vi "Transfer_function_diagonal_2register.vi"(0 "X reference":fxp<+/-,32,16>, 1 "Y reference":fxp<+/-,32,16>, 2 "Z reference":fxp<+/-,32,16>, 3 "X actual":fxp<+/-,33,17>, 4 "Y actual":fxp<+/-,33,17>, 5 "Z actual":fxp<+/-,33,17>, 6 "Scaling mV to V":fxp<+,33,10>=0.0009765625, 7 "xx1 Transfer Function":T1={"sos gain SF Controller"=0.0, "-a01(2)"=[0.0, 0.0, 0.0, 0.0, 0.0, 0.0, 0.0, 0.0, 0.0, 0.0, 0.0, 0.0, 0.0, 0.0, 0.0, 0.0, 0.0, 0.0, 0.0, 0.0], "-a02(2)"=[0.0, 0.0, 0.0, 0.0, 0.0, 0.0, 0.0, 0.0, 0.0, 0.0, 0.0, 0.0, 0.0, 0.0, 0.0, 0.0, 0.0, 0.0, 0.0, 0.0], "b01(2)"=[0.0, 0.0, 0.0, 0.0, 0.0, 0.0, 0.0, 0.0, 0.0, 0.0, 0.0, 0.0, 0.0, 0.0, 0.0, 0.0, 0.0, 0.0, 0.0, 0.0], "b02(2)"=[0.0, 0.0, 0.0, 0.0, 0.0, 0.0, 0.0, 0.0, 0.0, 0.0, 0.0, 0.0, 0.0, 0.0, 0.0, 0.0, 0.0, 0.0, 0.0, 0.0]}, 8 "Action":T2, 9 "yy1 Transfer Function":T1={"sos gain SF Controller"=0.0, "-a01(2)"=[0.0, 0.0, 0.0, 0.0, 0.0, 0.0, 0.0, 0.0, 0.0, 0.0, 0.0, 0.0, 0.0, 0.0, 0.0, 0.0, 0.0, 0.0, 0.0, 0.0], "-a02(2)"=[0.0, 0.0, 0.0, 0.0, 0.0, 0.0, 0.0, 0.0, 0.0, 0.0, 0.0, 0.0, 0.0, 0.0, 0.0, 0.0, 0.0, 0.0, 0.0, 0.0], "b01(2)"=[0.0, 0.0, 0.0, 0.0, 0.0, 0.0, 0.0, 0.0, 0.0, 0.0, 0.0, 0.0, 0.0, 0.0, 0.0, 0.0, 0.0, 0.0, 0.0, 0.0], "b02(2)"=[0.0, 0.0, 0.0, 0.0, 0.0, 0.0, 0.0, 0.0, 0.0, 0.0, 0.0, 0.0, 0.0, 0.0, 0.0, 0.0, 0.0, 0.0, 0.0, 0.0]}, 11 "zz1 Transfer Function":T1={"sos gain SF Controller"=0.0, "-a01(2)"=[0.0, 0.0, 0.0, 0.0, 0.0, 0.0, 0.0, 0.0, 0.0, 0.0, 0.0, 0.0, 0.0, 0.0, 0.0, 0.0, 0.0, 0.0, 0.0, 0.0], "-a02(2)"=[0.0, 0.0, 0.0, 0.0, 0.0, 0.0, 0.0, 0.0, 0.0, 0.0, 0.0, 0.0, 0.0, 0.0, 0.0, 0.0, 0.0, 0.0, 0.0, 0.0], "b01(2)"=[0.0, 0.0, 0.0, 0.0, 0.0, 0.0, 0.0, 0.0, 0.0, 0.0, 0.0, 0.0, 0.0, 0.0, 0.0, 0.0, 0.0, 0.0, 0.0, 0.0], "b02(2)"=[0.0, 0.0, 0.0, 0.0, 0.0, 0.0, 0.0, 0.0, 0.0, 0.0, 0.0, 0.0, 0.0, 0.0, 0.0, 0.0, 0.0, 0.0, 0.0, 0.0]}) -> (14 "X-stage voltage":fxp<+/-,32,16>, 15 "Y-stage voltage":fxp<+/-,32,16>, 16 "Z-stage voltage":fxp<+/-,32,16>, 17 "Kxx Output, Kxx*ex (V)":fxp<+/-,58,25>, 18 "Kyy Output, Kyy*ey (V)":fxp<+/-,58,25>, 19 "Kzz Output, Kzz*ez (V)":fxp<+/-,58,25>)   [LabVIEW 2015]
uses:
  Transfer_function_actions.ctl
  Transfer_function_coeffs.ctl
  <vilib>/rvi/Emulation/niFpgaGetClockAttributes.vi
  <vilib>/rvi/Emulation/niFpgaSctlEmulationGetInTimedLoop.vi
  <vilib>/rvi/Emulation/niFpgaEmulationReportErrorSimple.vi
  <vilib>/rvi/Emulation/niFpgaCriticalErrorInLSC.vi
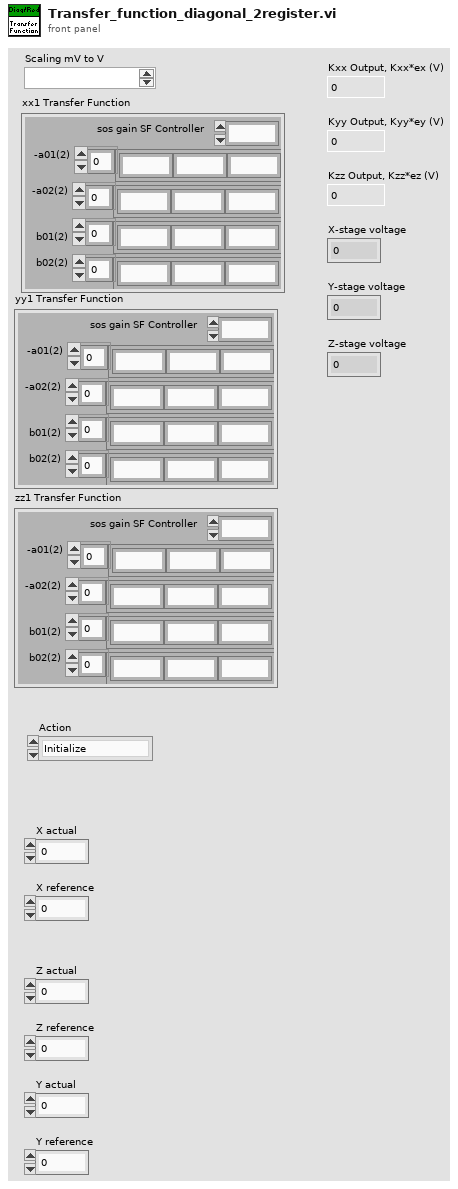
[diagram p1: front panel]
types:
  T1 = typedef "Transfer_function_coeffs.ctl" = cluster{"sos gain SF Controller":fxp<+/-,42,9>, "-a01(2)":fxp<+/-,64,9>[], "-a02(2)":fxp<+/-,64,9>[], "b01(2)":fxp<+/-,64,9>[], "b02(2)":fxp<+/-,64,9>[]}
  T2 = typedef "Transfer_function_actions.ctl" = enum16{"Initialize", "Calculate"}
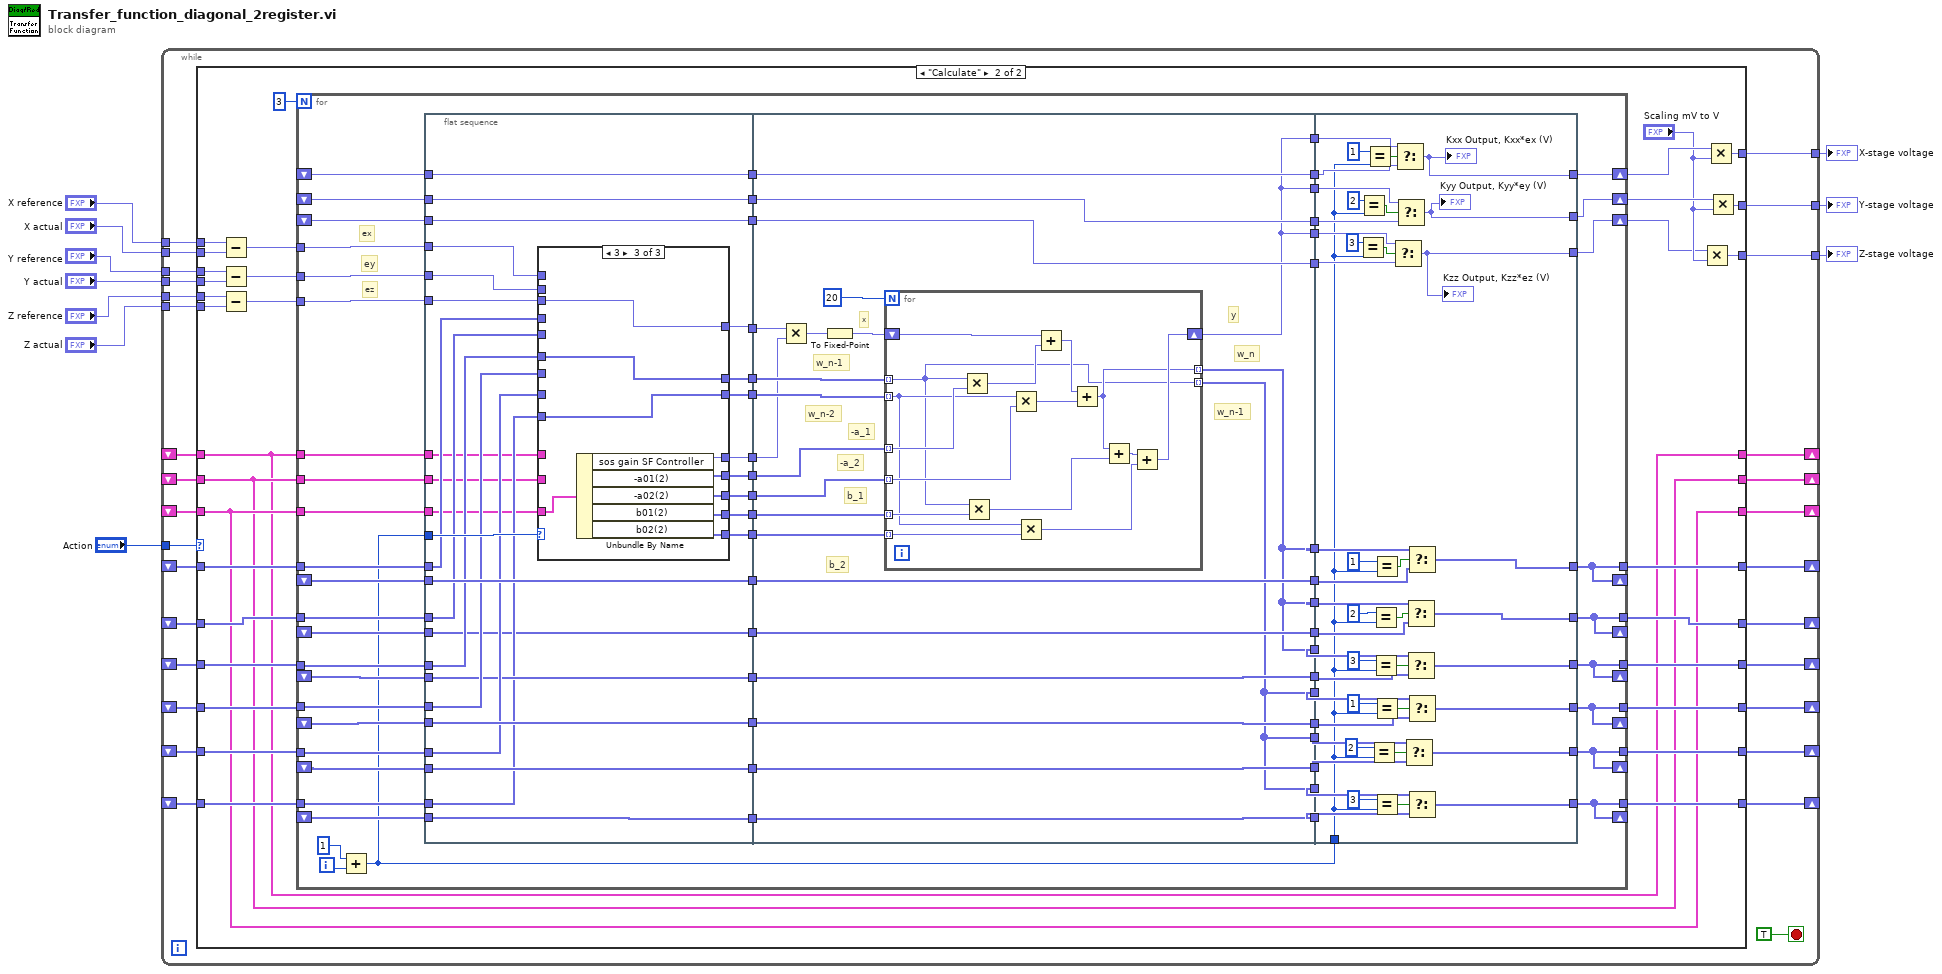
[diagram p0: block diagram]
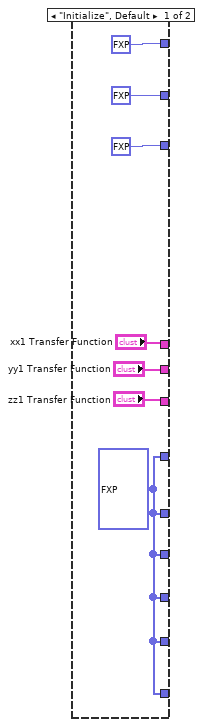
[diagram p2: hidden frame]
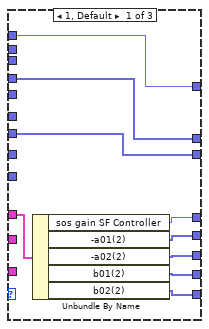
[diagram p3: hidden frame]
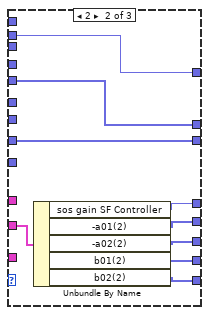
[diagram p4: hidden frame]
diagram:
  n1 = while {
    tunnel: [w39] -> w10
    tunnel: [w38] -> w9
    tunnel: [w37] -> w8
    tunnel: "Z reference" -> [w36]
    tunnel: "Y reference" -> [w35]
    tunnel: "X reference" -> [w34]
    tunnel: "Z actual" -> [w33]
    tunnel: "Y actual" -> [w32]
    tunnel: "X actual" -> [w31]
    shift-right: [w30] -> _
    shift-left: _ -> [w24]
    shift-right: [w29] -> _
    shift-left: _ -> [w23]
    shift-right: [w28] -> _
    shift-left: _ -> [w22]
    shift-right: [w27] -> _
    shift-left: _ -> [w21]
    shift-right: [w26] -> _
    shift-left: _ -> [w20]
    shift-right: [w25] -> _
    shift-left: _ -> [w19]
    tunnel: "Action" -> [w17]
    shift-right: [w13] -> _
    shift-left: _ -> [w16]
    shift-right: [w12] -> _
    shift-left: _ -> [w15]
    shift-right: [w11] -> _
    shift-left: _ -> [w14]
    stop <- TRUE stop-if-true
    n2 = case shown="\"Calculate\"" w17 {
      tunnel: [fxp<+/-,32,16> 0.0 w78] -> w39
      tunnel: [fxp<+/-,32,16> 0.0 w77] -> w38
      tunnel: [fxp<+/-,32,16> 0.0 w76] -> w37
      tunnel: w36 -> [_ w75]
      tunnel: w35 -> [_ w74]
      tunnel: w34 -> [_ w73]
      tunnel: w33 -> [_ w69]
      tunnel: w32 -> [_ w68]
      tunnel: w31 -> [_ w67]
      tunnel: [w43 w65] -> w30
      tunnel: [w43 w64] -> w29
      tunnel: [w43 w63] -> w28
      tunnel: [w43 w62] -> w27
      tunnel: [w43 w61] -> w26
      tunnel: [w43 w60] -> w25
      tunnel: w24 -> [_ w59]
      tunnel: w23 -> [_ w58]
      tunnel: w22 -> [_ w57]
      tunnel: w21 -> [_ w56]
      tunnel: w20 -> [_ w55]
      tunnel: w19 -> [_ w54]
      tunnel: w16 -> [_ w51]
      tunnel: w15 -> [_ w52]
      tunnel: w14 -> [_ w53]
      tunnel: ["xx1 Transfer Function" w51] -> w13
      tunnel: ["yy1 Transfer Function" w52] -> w12
      tunnel: ["zz1 Transfer Function" w53] -> w11
      frame "Initialize", Default {
        w43 = fxp<+/-,58,25>[] [0.0, 0.0, 0.0, 0.0, 0.0, 0.0, 0.0, 0.0, 0.0, 0.0, 0.0, 0.0, 0.0, 0.0, 0.0, 0.0, 0.0, 0.0, 0.0, 0.0]
      }
      frame "Calculate" {
        n3 = Subtract(x=w73, y=w67) -> (x-y=w50:fxp<+/-,58,25>)
        n4 = Subtract(x=w74, y=w68) -> (x-y=w49:fxp<+/-,58,25>)
        n5 = Subtract(x=w75, y=w69) -> (x-y=w48:fxp<+/-,58,25>)
        n6 = for {
          N: 3 -> [_]
          shift-right: [w132] -> w71
          shift-left: _ -> [w130]
          shift-right: [w129] -> w72
          shift-left: _ -> [w127]
          tunnel: [w84] -> w65
          shift-right: [w84] -> _
          shift-left: _ -> [w121]
          tunnel: [w83] -> w64
          shift-right: [w83] -> _
          shift-left: _ -> [w119]
          tunnel: w59 -> [w116]
          tunnel: w58 -> [w115]
          tunnel: [w81] -> w62
          shift-right: [w81] -> _
          shift-left: _ -> [w114]
          tunnel: [w80] -> w61
          shift-right: [w80] -> _
          shift-left: _ -> [w113]
          tunnel: w56 -> [w112]
          tunnel: w55 -> [w111]
          tunnel: w50 -> [w106]
          tunnel: w49 -> [w105]
          shift-right: [w104] -> w47
          shift-left: _ -> [w101]
          tunnel: [w82] -> w63
          tunnel: [w79] -> w60
          shift-right: [w82] -> _
          shift-left: _ -> [w96]
          shift-right: [w79] -> _
          shift-left: _ -> [w94]
          tunnel: w57 -> [w93]
          tunnel: w54 -> [w92]
          tunnel: w48 -> [w89]
          tunnel: w51 -> [w87]
          tunnel: w52 -> [w86]
          tunnel: w53 -> [w85]
          i -> [w137]
          # "ez"
          # "ey"
          # "ex"
          n7 = Add(x=1, y=w137) -> (x+y=w88:i32)
          n8 = flat-sequence {
            tunnel: [w175] -> w146
            tunnel: [w174] -> w145
            tunnel: [w173] -> w144
            tunnel: [w172] -> w143
            tunnel: [w171] -> w142
            tunnel: [w170] -> w141
            tunnel: [w169] -> w140
            tunnel: w88 -> [w176]
            tunnel: [w159] -> w139
            tunnel: [w168] -> w131
            tunnel: w130 -> [w168]
            tunnel: [w167] -> w128
            tunnel: w127 -> [w167]
            tunnel: [w166] -> w122
            tunnel: w121 -> [w166]
            tunnel: [w153] -> w120
            tunnel: w119 -> [w153]
            tunnel: w116 -> [w160]
            tunnel: w115 -> [w161]
            tunnel: w114 -> [w165]
            tunnel: w113 -> [w164]
            tunnel: w112 -> [w162]
            tunnel: w111 -> [w163]
            tunnel: [w165] -> w110
            tunnel: [w164] -> w109
            tunnel: w106 -> [w152]
            tunnel: w105 -> [w151]
            tunnel: [w158] -> w102
            tunnel: w101 -> [w158]
            tunnel: [w157] -> w97
            tunnel: w96 -> [w157]
            tunnel: [w156] -> w95
            tunnel: w94 -> [w156]
            tunnel: w93 -> [w154]
            tunnel: w92 -> [w155]
            tunnel: w89 -> [w150]
            tunnel: w87 -> [w149]
            tunnel: w86 -> [w148]
            tunnel: w85 -> [w147]
            tunnel: w146 -> [w224]
            tunnel: w145 -> [w223]
            tunnel: w144 -> [w208]
            tunnel: w143 -> [w209]
            tunnel: w142 -> [w210]
            tunnel: w141 -> [w211]
            tunnel: w140 -> [w212]
            tunnel: w139 -> [w215]
            tunnel: [w204] -> w136
            tunnel: [w204] -> w135
            tunnel: [w206] -> w134
            tunnel: [w207] -> w133
            tunnel: w131 -> [w207]
            tunnel: w128 -> [w206]
            tunnel: [w214] -> w126
            tunnel: [w214] -> w125
            tunnel: [w213] -> w124
            tunnel: [w213] -> w123
            tunnel: w122 -> [w222]
            tunnel: w120 -> [w221]
            tunnel: [w222] -> w118
            tunnel: [w221] -> w117
            tunnel: w110 -> [w220]
            tunnel: w109 -> [w219]
            tunnel: [w220] -> w108
            tunnel: [w219] -> w107
            tunnel: [w204] -> w103
            tunnel: w102 -> [w218]
            tunnel: [w218] -> w100
            tunnel: [w214] -> w99
            tunnel: [w213] -> w98
            tunnel: w97 -> [w217]
            tunnel: w95 -> [w216]
            tunnel: [w217] -> w91
            tunnel: [w216] -> w90
            tunnel: w136 -> [w244]
            tunnel: w135 -> [w283]
            tunnel: w88 -> [w243]
            tunnel: w134 -> [w282]
            tunnel: w133 -> [w245]
            tunnel: [w242] -> w132
            tunnel: [w247] -> w129
            tunnel: w126 -> [w273]
            tunnel: w125 -> [w272]
            tunnel: w124 -> [w271]
            tunnel: w123 -> [w270]
            tunnel: [w269] -> w84
            tunnel: [w268] -> w83
            tunnel: w118 -> [w267]
            tunnel: w117 -> [w266]
            tunnel: [w265] -> w81
            tunnel: [w264] -> w80
            tunnel: w108 -> [w263]
            tunnel: w107 -> [w262]
            tunnel: [w246] -> w104
            tunnel: w103 -> [w259]
            tunnel: w100 -> [w258]
            tunnel: w99 -> [w253]
            tunnel: w98 -> [w252]
            tunnel: [w251] -> w82
            tunnel: [w250] -> w79
            tunnel: w91 -> [w249]
            tunnel: w90 -> [w248]
            frame #0 {
              n9 = case shown="3" w176 {
                tunnel: [w182 w190 w199] -> w173
                tunnel: [w181 w189 w198] -> w172
                tunnel: [w180 w188 w197] -> w171
                tunnel: [w179 w187 w196] -> w170
                tunnel: [w178 w186 w195] -> w169
                tunnel: [w183 w193 w202] -> w174
                tunnel: [w184 w192 w201] -> w175
                tunnel: w160 -> [w184 _ _]
                tunnel: w161 -> [_ w192 _]
                tunnel: w162 -> [w183 _ _]
                tunnel: w163 -> [_ w193 _]
                tunnel: [w185 w194 w203] -> w159
                tunnel: w152 -> [w185 _ _]
                tunnel: w151 -> [_ w194 _]
                tunnel: w155 -> [_ _ w202]
                tunnel: w154 -> [_ _ w201]
                tunnel: w150 -> [_ _ w203]
                tunnel: w149 -> [w177 _ _]
                tunnel: w148 -> [_ w191 _]
                tunnel: w147 -> [_ _ w200]
                frame 1, Default {
                  n10 = Unbundle By Name(w177) -> ("sos gain SF Controller"=w182:fxp<+/-,42,9>, "-a01(2)"=w181:fxp<+/-,64,9>[], "-a02(2)"=w180:fxp<+/-,64,9>[], "b01(2)"=w179:fxp<+/-,64,9>[], "b02(2)"=w178:fxp<+/-,64,9>[])
                }
                frame 2 {
                  n11 = Unbundle By Name(w191) -> ("sos gain SF Controller"=w190:fxp<+/-,42,9>, "-a01(2)"=w189:fxp<+/-,64,9>[], "-a02(2)"=w188:fxp<+/-,64,9>[], "b01(2)"=w187:fxp<+/-,64,9>[], "b02(2)"=w186:fxp<+/-,64,9>[])
                }
                frame 3 {
                  n12 = Unbundle By Name(w200) -> ("sos gain SF Controller"=w199:fxp<+/-,42,9>, "-a01(2)"=w198:fxp<+/-,64,9>[], "-a02(2)"=w197:fxp<+/-,64,9>[], "b01(2)"=w196:fxp<+/-,64,9>[], "b02(2)"=w195:fxp<+/-,64,9>[])
                }
              }
            }
            frame #1 {
              # "b_2"
              # "b_1"
              # "-a_2"
              # "-a_1"
              # "w_n-2"
              # "x"
              # "w_n-1"
              # "w_n-1"
              # "w_n"
              # "y"
              n13 = Multiply(x=w215, y=w208) -> (x*y=w225:fxp<+/-,64,34>)
              n14 = To Fixed-Point(number=w225) -> (fixed-point=w226:fxp<+/-,58,25>)  [unwired: 1 in]
              n15 = for {
                N: 20 -> [_]
                tunnel: w209 -> [w240] mode=indexing
                tunnel: w212 -> [w235] mode=indexing
                shift-right: [w232] -> w204
                shift-left: w226 -> [w241]
                tunnel: w210 -> [w236] mode=indexing
                tunnel: w211 -> [w239] mode=indexing
                tunnel: [w229] -> w214 mode=indexing
                tunnel: w224 -> [w227] mode=indexing
                tunnel: [w227] -> w213 mode=indexing
                tunnel: w223 -> [w234] mode=indexing
                n16 = Multiply(x=w227, y=w240) -> (x*y=w228:fxp<+/-,58,25>)
                n17 = Multiply(x=w227, y=w239) -> (x*y=w231:fxp<+/-,58,25>)
                n18 = Multiply(x=w234, y=w236) -> (x*y=w230:fxp<+/-,58,25>)
                n19 = Multiply(x=w234, y=w235) -> (x*y=w233:fxp<+/-,58,25>)
                n20 = Add(x=w241, y=w228) -> (x+y=w238:fxp<+/-,58,25>)
                n21 = Add(x=w238, y=w230) -> (x+y=w229:fxp<+/-,58,25>)
                n22 = Add(x=w229, y=w231) -> (x+y=w237:fxp<+/-,58,25>)
                n23 = Add(x=w237, y=w233) -> (x+y=w232:fxp<+/-,58,25>)
              }
            }
            frame #2 {
              n24 = Equal?(x=3, y=w243) -> (x = y?=w260:bool)
              n25 = Equal?(x=2, y=w243) -> (x = y?=w284:bool)
              n26 = Equal?(x=1, y=w243) -> (x = y?=w286:bool)
              n27 = Equal?(x=2, y=w243) -> (x = y?=w274:bool)
              n28 = Equal?(x=2, y=w243) -> (x = y?=w278:bool)
              n29 = Equal?(x=3, y=w243) -> (x = y?=w256:bool)
              n30 = Equal?(x=1, y=w243) -> (x = y?=w280:bool)
              n31 = Equal?(x=1, y=w243) -> (x = y?=w276:bool)
              n32 = Equal?(x=3, y=w243) -> (x = y?=w254:bool)
              n33 = Select(t=w259, s=w260, f=w258) -> (s? t:f=w246:fxp<+/-,58,25>)
              "Kzz Output, Kzz*ez (V)" <- w246
              n34 = Select(t=w244, s=w286, f=w245) -> (s? t:f=w242:fxp<+/-,58,25>)
              "Kxx Output, Kxx*ex (V)" <- w242
              n35 = Select(t=w283, s=w284, f=w282) -> (s? t:f=w247:fxp<+/-,58,25>)
              "Kyy Output, Kyy*ey (V)" <- w247
              n36 = Select(t=w270, s=w274, f=w262) -> (s? t:f=w264:fxp<+/-,58,25>[])
              n37 = Select(t=w272, s=w278, f=w266) -> (s? t:f=w268:fxp<+/-,58,25>[])
              n38 = Select(t=w253, s=w256, f=w249) -> (s? t:f=w251:fxp<+/-,58,25>[])
              n39 = Select(t=w273, s=w280, f=w267) -> (s? t:f=w269:fxp<+/-,58,25>[])
              n40 = Select(t=w271, s=w276, f=w263) -> (s? t:f=w265:fxp<+/-,58,25>[])
              n41 = Select(t=w252, s=w254, f=w248) -> (s? t:f=w250:fxp<+/-,58,25>[])
            }
          }
        }
        n42 = Multiply(x=w47, y="Scaling mV to V") -> (x*y=w77:fxp<+/-,32,16>)
        n43 = Multiply(x=w71, y="Scaling mV to V") -> (x*y=w78:fxp<+/-,32,16>)
        n44 = Multiply(x=w72, y="Scaling mV to V") -> (x*y=w76:fxp<+/-,32,16>)
      }
    }
  }
  "X-stage voltage" <- w10
  "Z-stage voltage" <- w9
  "Y-stage voltage" <- w8
